vi "Find Post-Setup Actors.vi"(11 "Actor in":refnum<class "Actor.lvclass">) -> (2 "Post-Setup Actors":refnum<class "Actor.lvclass">[](array[class]))   [LabVIEW 2020, in "jettl.lvlib" / "Actor.lvclass"]
uses:
  Actor.lvclass
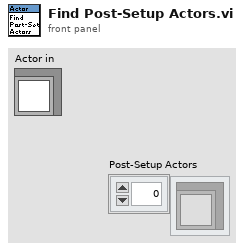
[diagram p1: front panel]
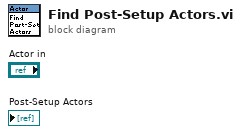
[diagram p0: block diagram]
diagram:
